vi "Puff_Dose_from_Continuous.vi"() -> (5 "Plug in titles":string[](array[string]), 7 "Plug in values":string[](array[string]))   [LabVIEW 2020]
uses:
  File/File Update Cluster.ctl
  Globals/Meas_global.vi
  Globals/Plug_in_data_global.vi
  <vilib>/Analysis/NI_AALBase.lvlib
panel:
  in  "File Extension":string=".xls"
  in  "Save Puff traces":bool
  in  "Gap between Puffs":dbl=0.25
  out "Dose per Sudo Puff":dbl[](graph)
  out "Concentration Trace":dbl[](graph)
  in  "Puff length (s)":dbl=0.25
  out "D'/Dmean":dbl
  out "St Dev of Dose":dbl format="%0.2f"
  out "Mean Dose":dbl format="%0.2f"
  # "Only Saves puff data\nif Saving results file"
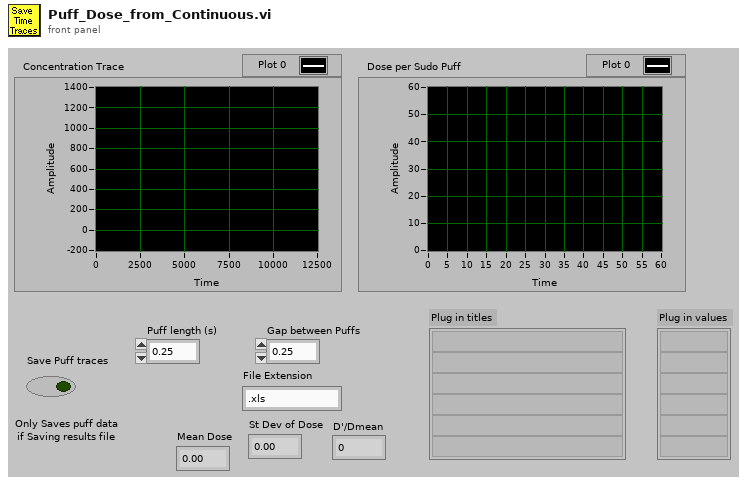
[diagram p1: front panel]
types:
  T1 = enum16{"Save no data", "Save data in new files", "Save data in existing files"}
  T2 = typedef "File Update Cluster.ctl" = cluster{"File Path":path, "Rows to Add":i32[], "Extra Ch Names":string[], "Extra Ch Values":string[], "Initial Header String":string, "Separation Character":enum16{"Tab", "Comma"}}
  T3 = typedef "Time_Trace_Cluster.ctl" = cluster{"Weighting":dbl[], "Time (s)":dbl[], "Voltage":dbl[], "Eng Values":dbl[]}
  T4 = typedef "Analysis_info_cluster.ctl" = cluster{"Colour":u32, "Inst type":T5, "Inst name":string, "Symbol":string, "Code name":string, "Extra Info":string, "Inst Array":T6, "Extra Titles":string[], "Extra Values":string[], "U":dbl, "u^2":dbl, "u^3":dbl, "u^4":dbl, "Skew_u":dbl, "Kurt_u":dbl, "Sd Error in Mean":dbl, "% u'/U":dbl, "X":dbl, "Y":dbl, "Z":dbl, "Timescale integral Estimate":dbl, "Sd Error in Variance":dbl, "Calib File":path, "Calib Constants":dbl[], "Output Position":bool, "Stats":enum16{"None", "Basic", "Full"}, "Av Sampling Rate":dbl, "Av No of Samples":dbl, "Total Meas Time (s)":dbl, "ADAM Ch Name":string, "Max value":dbl, "Min value":dbl, "Req Sample Rate Hz":dbl, "Sync Delay Time (s)":dbl, "Ch No":i16, "Device":string, "Use Latest Calib":bool, "Port":string, "Metadata Ch Names":string[], "Metadata Ch Values":string[]}
  T5 = typedef "Inst_type.ctl" = enum16{"Propeller anemometer", "Raw voltage", "Pressure Transducer", "Pitot-static tube", "Preston tube", "Hot wire", "Cross wire 1", "Cross wire 2", "Generic Linear", "Generic Polynomial", "Generic BackPoly", "Fast FID", "Thermocouple", "Cold wire", "Pulsed Wire", "LDA Vel", "LDA Tran time", "LDA Arr time", "Microphone"}
  T6 = typedef "Instrument_Array.ctl" = enum16{"PWA", "LDA", "Analogue"}
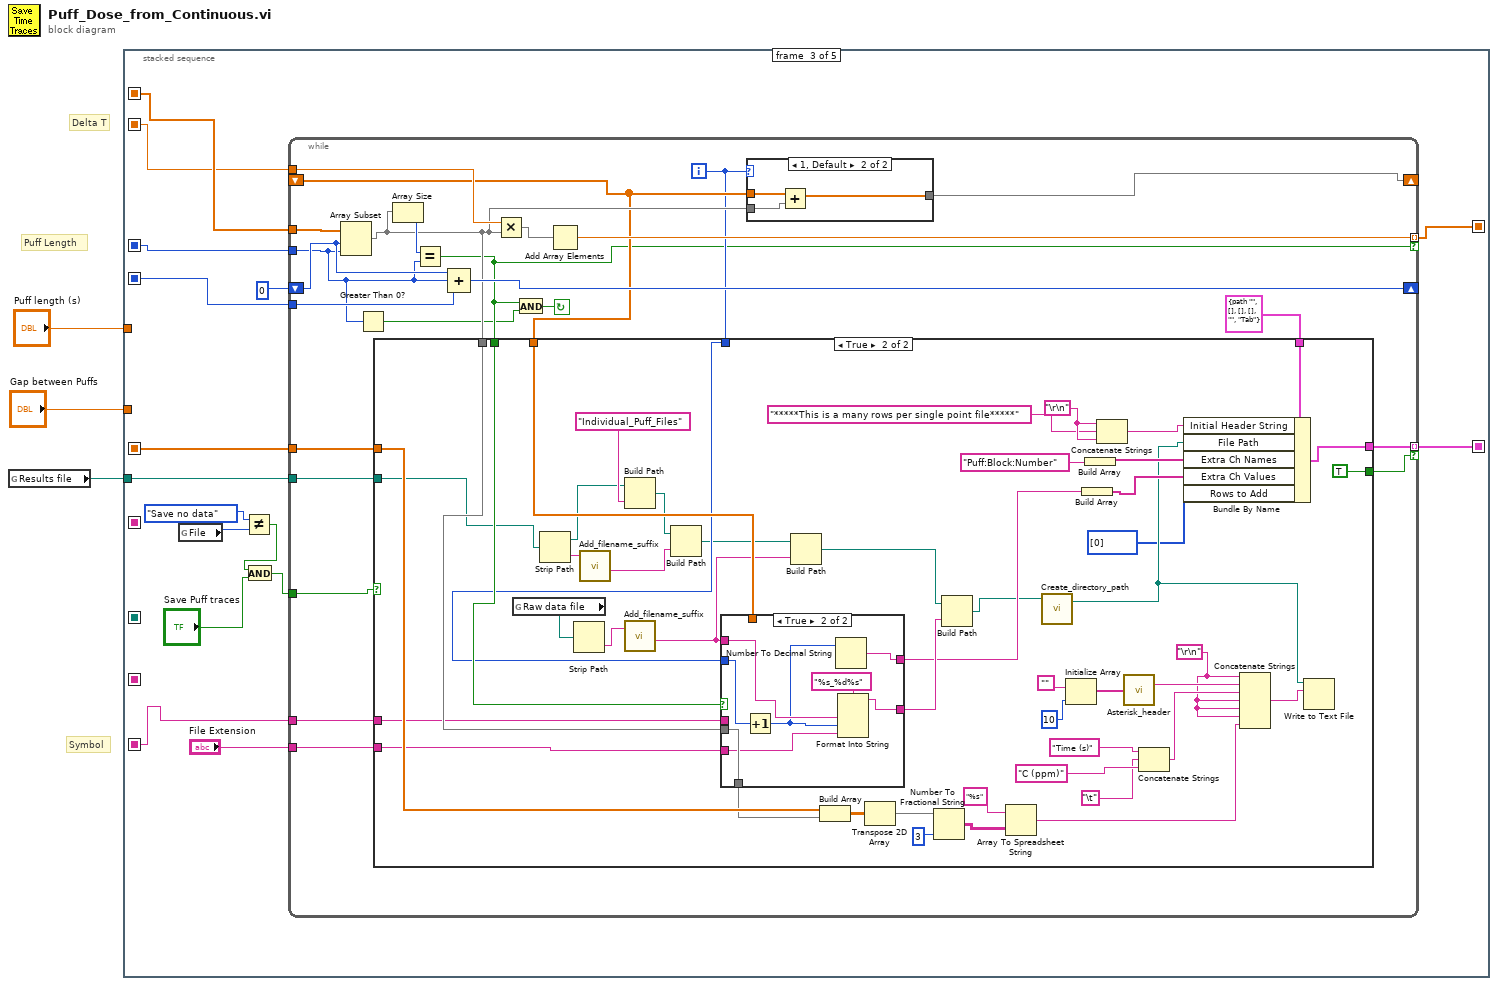
[diagram p0: block diagram]
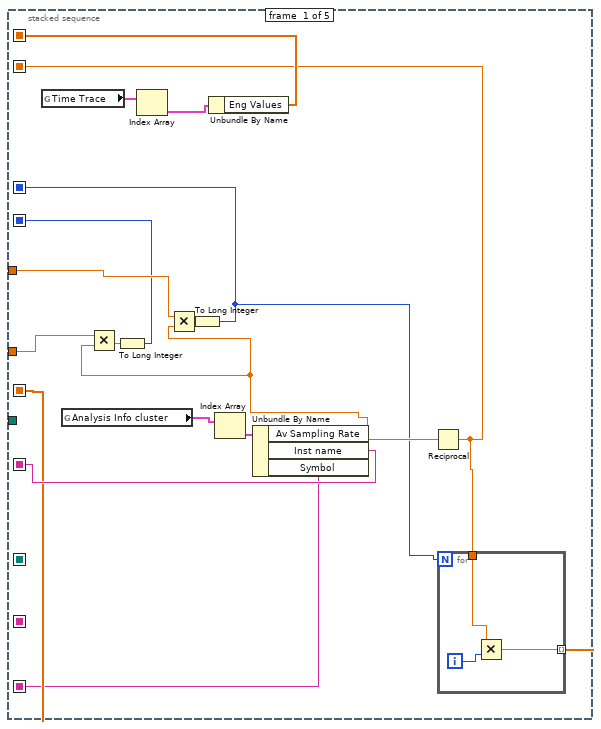
[diagram p2: hidden frame]
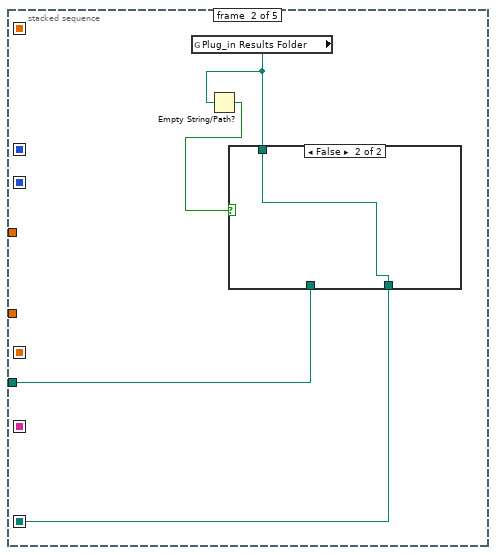
[diagram p3: hidden frame]
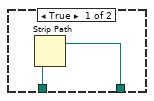
[diagram p4: hidden frame]
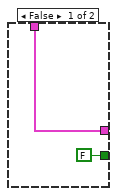
[diagram p6: hidden frame]
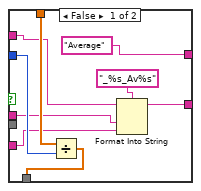
[diagram p7: hidden frame]
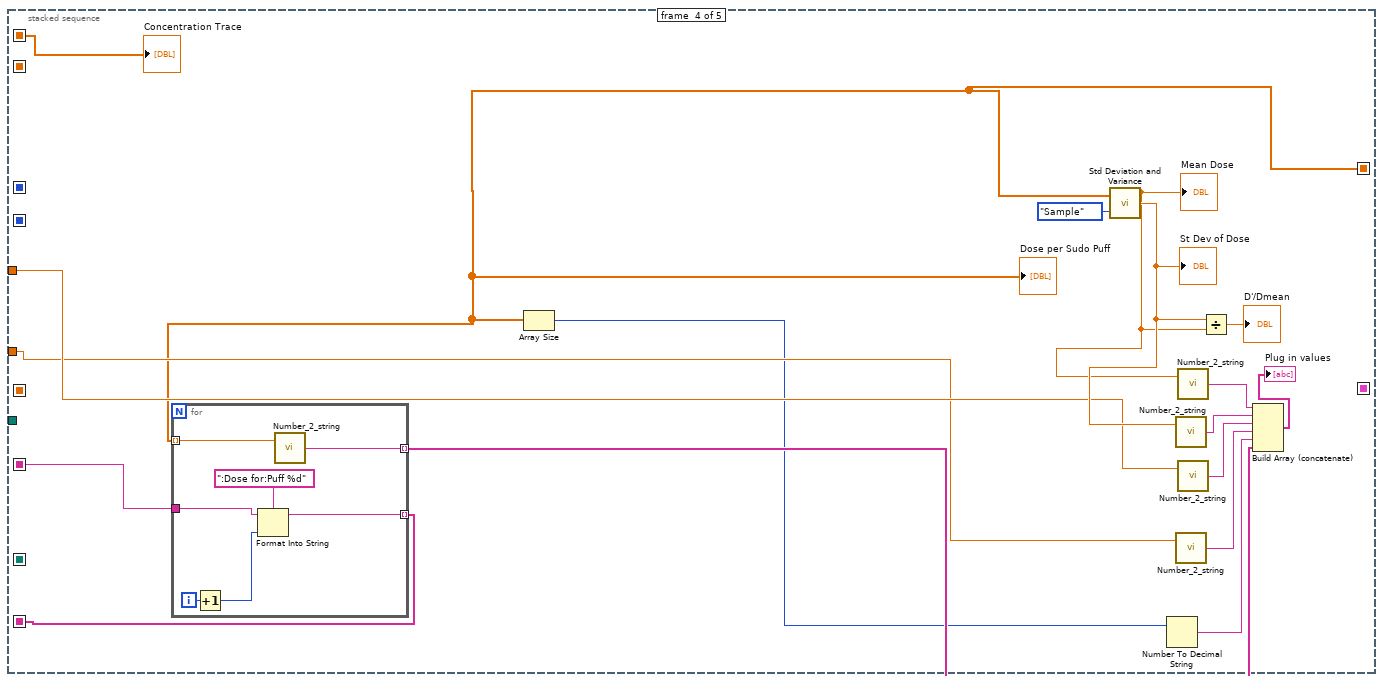
[diagram p8: hidden frame]
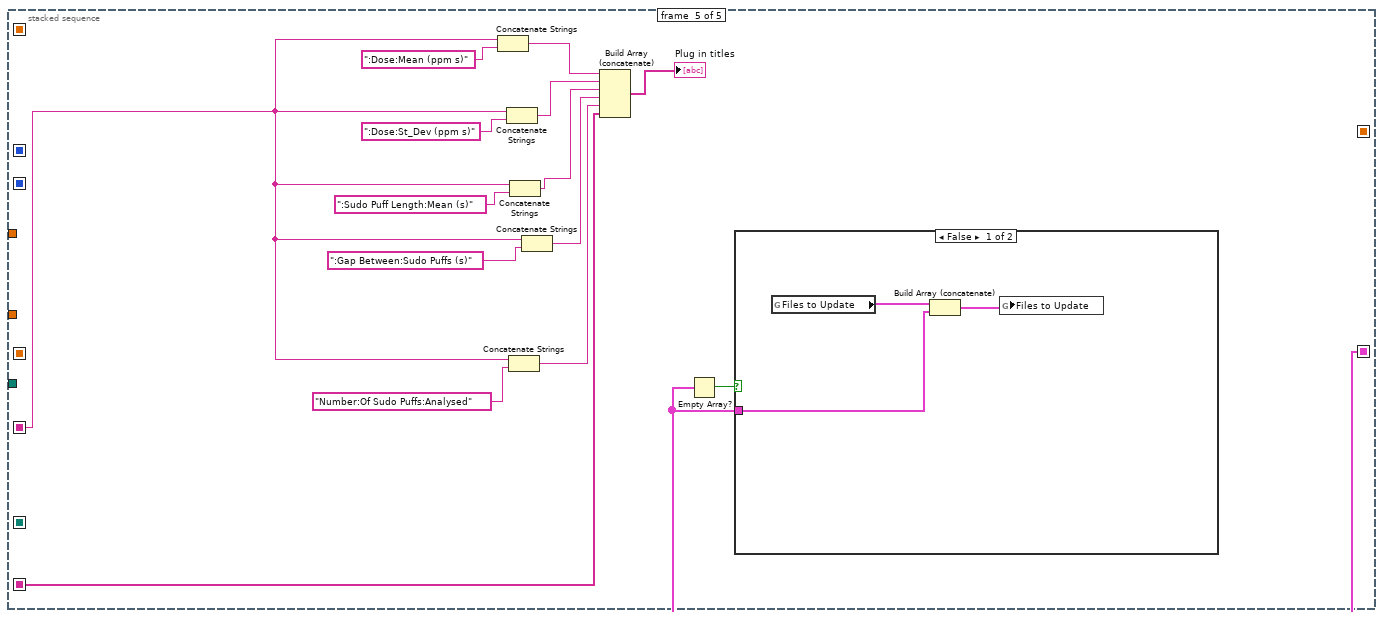
[diagram p9: hidden frame]
diagram:
  # "Symbol"
  # "Delta T"
  # "Puff Length"
  n1 = global read "Meas_global.vi" "Results file"() -> (w1:path)
  n2 = stacked-sequence {
    seq-local: [w15 _ _ _ _] -> [_ _ _ w150 w170]
    seq-local: [w8 _ _ _ _] -> [_ _ w44 w143 _]
    seq-local: [w7 _ _ _ _] -> [_ _ w45 _ _]
    seq-local: [_ _ _ w149 _] -> [_ _ _ _ w167]
    seq-local: [w9 _ _ _ _] -> [_ _ w42 _ _]
    seq-local: [w6 _ _ _ _] -> [_ _ w41 _ _]
    seq-local: [w5 _ _ _ _] -> [_ _ w40 _ _]
    seq-local: [_ w24 _ _ _] -> [_ _ _ _ _]
    seq-local: [w4 _ _ _ _] -> [_ _ w37 _ _]
    seq-local: [_ _ w36 _ _] -> [_ _ _ _ w173]
    seq-local: [_ _ w35 _ _] -> [_ _ _ w142 _]
    tunnel: "Puff length (s)" -> [w13 _ _ w152 _]
    tunnel: "Gap between Puffs" -> [w11 _ _ w147 _]
    tunnel: w1 -> [_ w23 w39 _ _]
    frame #0 {
      n3 = global read "Meas_global.vi" "Time Trace"() -> (w19:T3[])
      n4 = global read "Meas_global.vi" "Analysis Info cluster"() -> (w17:T4[])
      n5 = Index Array(array=w19) -> (element=w18:T3)  [unwired: 1 in]
      n6 = Unbundle By Name(w18) -> ("Eng Values"=w8:dbl[])
      n7 = Index Array(array=w17) -> (element=w16:T4)  [unwired: 1 in]
      n8 = Unbundle By Name(w16) -> ("Av Sampling Rate"=w12:dbl, "Inst name"=w15:string, "Symbol"=w4:string)
      n9 = Multiply(x=w11, y=w12) -> (x*y=w10:dbl)
      n10 = To Long Integer(number=w10) -> (32bit integer=w9:i32)
      n11 = Multiply(x=w13, y=w12) -> (x*y=w14:dbl)
      n12 = To Long Integer(number=w14) -> (32bit integer=w7:i32)
      n13 = Reciprocal(x=w12) -> (1/x=w6:dbl)
      n14 = for {
        N: w7 -> [_]
        tunnel: w6 -> [w21]
        tunnel: [w20] -> w5 mode=indexing
        i -> [w22]
        n15 = Multiply(x=w21, y=w22) -> (x*y=w20:dbl)
      }
    }
    frame #1 {
      n16 = global read "Plug_in_data_global.vi" "Plug_in Results Folder"() -> (w26:path)
      n17 = Empty String/Path?(string/path=w26) -> (empty?=w25:bool)
      n18 = case shown="False" w25 {
        tunnel: w26 -> [_ w29]
        tunnel: [w28 w29] -> w24
        tunnel: w23 -> [w27 _]
        frame True {
          n19 = Strip Path(path=w27) -> (stripped path=w28:path)  [unwired: 1 out]
        }
        frame False {
        }
      }
    }
    frame #2 {
      n20 = global read "Meas_global.vi" "File"() -> (w33:T1)
      n21 = Not Equal?(x=T1."Save no data" ("File"), y=w33) -> (x != y?=w32:bool)
      n22 = And(x=w32, y="Save Puff traces") -> (x .and. y?=w30:bool)
      n23 = while {
        tunnel: w44 -> [w69]
        tunnel: w45 -> [w49]
        tunnel: [w68] -> w35 mode=indexing if=w48
        shift-right: [w65] -> _
        shift-left: 0 -> [w67]
        tunnel: w42 -> [w66]
        tunnel: w41 -> [w62]
        tunnel: w40 -> [w61]
        tunnel: w30 -> [w60]
        shift-right: [w59] -> _
        shift-left: _ -> [w57]
        tunnel: w39 -> [w55]
        tunnel: "File Extension" -> [w54]
        tunnel: w37 -> [w53]
        tunnel: [w52] -> w36 mode=indexing if=w50
        i -> [w56]
        stop <- w46 continue-if-true
        n24 = Array Subset(array=w69, index=w67, length=w49) -> (w58:dbl[])
        n25 = Greater Than 0?(x=w49) -> (x > 0?=w47:bool)
        n26 = Array Size(array=w58) -> (size(s)=w64:i32)
        n27 = Equal?(x=w64, y=w49) -> (x = y?=w48:bool)
        n28 = case shown="True" w60 {
          tunnel: w61 -> [_ w121]
          tunnel: w58 -> [_ w118]
          tunnel: w48 -> [_ w120]
          tunnel: w57 -> [_ w117]
          tunnel: w56 -> [_ w116]
          tunnel: w55 -> [_ w102]
          tunnel: w54 -> [_ w108]
          tunnel: w53 -> [_ w105]
          tunnel: [w75 w80] -> w52
          tunnel: T2 {"File Path"=path "", "Rows to Add"=[], "Extra Ch Names"=[], "Extra Ch Values"=[], "Initial Header String"="", "Separation Character"=enum."Tab"} ("File to Update") -> [w75 w79]
          tunnel: [FALSE TRUE] -> w50
          frame False {
          }
          frame True {
            w84 = "\r\n"
            w110 = "\r\n"
            n29 = global read "Meas_global.vi" "Raw data file"() -> (w107:path)
            n30 = Strip Path(path=w102) -> (stripped path=w76:path, name=w103:string)
            n31 = Strip Path(path=w107) -> (name=w106:string)  [unwired: 1 out]
            n32 = call "Add_filename_suffix.vi"("Filename"=w103) -> ("Base name"=w100:string)  [unwired: 1 in, 3 out]
            n33 = Build Path(base path=w76, name or relative path="Individual_Puff_Files") -> (appended path=w101:path)
            n34 = call "Add_filename_suffix.vi"("Filename"=w106) -> ("Base name"=w98:string)  [unwired: 1 in, 3 out]
            n35 = Build Path(base path=w101, name or relative path=w100) -> (appended path=w99:path)
            n36 = case shown="True" w120 {
              tunnel: [w131 w141] -> w119
              tunnel: w118 -> [_ w141]
              tunnel: w117 -> [w133 _]
              tunnel: w116 -> [w132 w139]
              tunnel: w108 -> [w128 w138]
              tunnel: w98 -> [w129 w137]
              tunnel: w105 -> [w127 _]
              tunnel: [w126 w136] -> w96
              tunnel: ["Average" w134] -> w94
              frame False {
                n37 = Divide(x=w133, y=w132) -> (x/y=w131:dbl[])
                n38 = Format Into String(format string="_%s_Av%s", initial string=w129, w127, w128) -> (resulting string=w126:string)  [unwired: 1 in, 1 out]
              }
              frame True {
                n39 = Increment(x=w139) -> (x+1=w135:i32)
                n40 = Number To Decimal String(number=w135) -> (decimal integer string=w134:string)  [unwired: 1 in]
                n41 = Format Into String(format string="%s_%d%s", w137, w135, w138) -> (resulting string=w136:string)  [unwired: 2 in, 1 out]
              }
            }
            n42 = Build Path(base path=w99, name or relative path=w98) -> (appended path=w97:path)
            n43 = Build Array(w121, w119) -> (w122:dbl[][])
            n44 = Transpose 2D Array(2D array=w122) -> (transposed array=w123:dbl[][])
            n45 = Number To Fractional String(number=w123, precision (6)=i16 3) -> (F-format string=w114:string[][])  [unwired: 2 in]
            n46 = Build Path(base path=w97, name or relative path=w96) -> (appended path=w93:path)
            n47 = Array To Spreadsheet String(array=w114, 3:"%s" ("format string")) -> (spreadsheet string=w83:string)  [unwired: 1 in]
            n48 = call "Create_directory_path.vi"("Path name"=w93) -> ("Path name Out"=w82:path)  [unwired: 2 in, 1 out]
            n49 = Initialize Array("", 10) -> (w87:string[])
            n50 = Build Array(w94) -> (w95:string[])
            n51 = Build Array("Puff:Block:Number" ("element")) -> (w113:string[])
            n52 = Concatenate Strings(w110, "*****This is a many rows per single point file*****", w110) -> (w111:string)
            n53 = call "Asterisk_header.vi"("Channel names"=w87) -> ("Header string"=w88:string)
            n54 = Concatenate Strings("Time (s)", "\t", "C (ppm)") -> (w92:string)
            n55 = Bundle By Name(cluster=w79, "Initial Header String"=w111, "File Path"=w82, "Extra Ch Names"=w113, "Extra Ch Values"=w95, "Rows to Add"=i32[] [0]) -> (w80:T2)
            n56 = Concatenate Strings(w84, w88, w92, w84, w84, w84, w83) -> (w81:string)
            n57 = Write to Text File(file (use dialog)=w82, text=w81) -> ()  [unwired: 2 in, 3 out]
          }
        }
        n58 = Compound Arithmetic op=ADD(w67, w49, w66) -> (w65:i32)
        n59 = Multiply(x=w62, y=w58) -> (x*y=w63:dbl[])
        n60 = And(x=w48, y=w47) -> (x .and. y?=w46:bool)
        n61 = Add Array Elements(numeric array=w63) -> (sum=w68:dbl)
        n62 = case shown="1, Default" w56 {
          tunnel: [w70 w71] -> w59
          tunnel: w58 -> [w70 w73]
          tunnel: w57 -> [_ w72]
          frame 0 {
          }
          frame 1, Default {
            n63 = Add(x=w72, y=w73) -> (x+y=w71:dbl[])
          }
        }
      }
    }
    frame #3 {
      n64 = for {
        tunnel: w142 -> [w166] mode=indexing
        tunnel: w150 -> [w164]
        tunnel: [w161] -> w148 mode=indexing
        tunnel: [w160] -> w149 mode=indexing
        i -> [w165]
        n65 = Increment(x=w165) -> (x+1=w162:i32)
        n66 = Format Into String(format string=":Dose for:Puff %d", initial string=w164, w162) -> (resulting string=w160:string)  [unwired: 1 in, 1 out]
        n67 = call "Number_2_string.vi"("number"=w166) -> ("String"=w161:string)  [unwired: 1 in]
      }
      n68 = Array Size(array=w142) -> (size(s)=w145:i32)
      n69 = call <vilib>:"Std Deviation and Variance.vi"("X"=w142, "Weighting (Sample)"=enum16{"Sample", "Population"}."Sample") -> ("mean"=w157:dbl, "standard deviation"=w158:dbl)  [unwired: 1 out]
      "Mean Dose" <- w157
      "St Dev of Dose" <- w158
      n70 = Number To Decimal String(number=w145) -> (decimal integer string=w144:string)  [unwired: 1 in]
      n71 = call "Number_2_string.vi"("number"=w158) -> ("String"=w154:string)  [unwired: 1 in]
      n72 = call "Number_2_string.vi"("number"=w147) -> ("String"=w146:string)  [unwired: 1 in]
      n73 = call "Number_2_string.vi"("number"=w157) -> ("String"=w155:string)  [unwired: 1 in]
      n74 = call "Number_2_string.vi"("number"=w152) -> ("String"=w151:string)  [unwired: 1 in]
      n75 = Divide(x=w158, y=w157) -> (x/y=→"D'/Dmean":dbl)
      n76 = Build Array (concatenate)(w155, w154, w151, w146, w144, w148) -> (→"Plug in values":string[])
      "Dose per Sudo Puff" <- w142
      "Concentration Trace" <- w143
    }
    frame #4 {
      n77 = Concatenate Strings(w170, ":Dose:Mean (ppm s)" ("string")) -> (w179:string)
      n78 = Concatenate Strings(w170, ":Dose:St_Dev (ppm s)" ("string")) -> (w180:string)
      n79 = Concatenate Strings(w170, "Number:Of Sudo Puffs:Analysed" ("format string")) -> (w168:string)
      n80 = Concatenate Strings(w170, ":Sudo Puff Length:Mean (s)" ("string")) -> (w175:string)
      n81 = Concatenate Strings(w170, ":Gap Between:Sudo Puffs (s)" ("string")) -> (w169:string)
      n82 = Build Array (concatenate)(w179, w180, w175, w169, w168, w167) -> (→"Plug in titles":string[])
      n83 = Empty Array?(array=w173) -> (empty?=w174:bool)
      n84 = case shown="False" w174 {
        tunnel: w173 -> [w183 _]
        frame False {
          n85 = global read "Meas_global.vi" "Files to Update"() -> (w184:T2[])
          n86 = Build Array (concatenate)(w184, w183) -> (w182:T2[])
          n87 = global write "Meas_global.vi" "Files to Update"(w182) -> ()
        }
        frame True {
        }
      }
    }
  }
